vi "Fractional-octave Analysis with IC (peak mode).vi"(0 "scaled signal [EU]":dbl[](array[numeric]) format="%.2f", 1 "peak detection mode":T1(ring), 2 "filter bank parameters":T2 {"standard filter bandwidth" format="%.2f"; "special filter bandwidth" format="%.2f"; "lowpass filter coefficients"."Forward Coefficients" format="%.2f"; "lowpass filter coefficients"."Reverse Coefficients" format="%.2f"; "standard filter coefficients"."Forward Coefficients" format="%.2f"; "standard filter coefficients"."Reverse Coefficients" format="%.2f"; "special filter coefficients"."Forward Coefficients" format="%.2f"; "special filter coefficients"."Reverse Coefficients" format="%.2f"}, 3 "internal filter state IN":T3 {"linear averaging"."size" format="%.2f"; "linear averaging"."squared sum" format="%.2f"; "exponential averaging"."peak detector" format="%.2f"; "exponential averaging"."exponential averaging" format="%.2f"; "result" format="%.2f"; "lowpass filter" format="%.2f"; "octave filter"."Octave filter" format="%.2f"}, 4 "reset peak detection (F)":bool, 5 "filter init/cont (init:F)":bool) -> (6 "peak band power [EU^2 rms]":dbl[](array[numeric]) format="%.2f", 7 "settled?":bool, 8 "internal filter state OUT":T3 {"linear averaging"."size" format="%.2f"; "linear averaging"."squared sum" format="%.2f"; "exponential averaging"."peak detector" format="%.2f"; "exponential averaging"."exponential averaging" format="%.2f"; "result" format="%.2f"; "lowpass filter" format="%.2f"; "octave filter"."Octave filter" format="%.2f"})   [LabVIEW 2017]
doc: "Performs a peak fractional-octave analysis on the input signal. This VI requires the filter bank parameters and initialize filter state information the Design Octave Filter Set VI generates.\nThis VI returns the peak power in each fractional-octave band.\nThe internal filter state IN and internal filter state OUT keep track of the internal state of the filter to ensure continuous operation of the filter. To achieve this continuous operation, you must call this VI the first time with filter init/cont set to FALSE. Call it all subsequent times with filter init/cont set to TRUE. Wire the internal filter state OUT of this call to the internal filter state IN for the next call to this VI."
uses:
  <vilib>/addons/Sound and Vibration/svt_Octave/SoundVib_Octave.lvlib
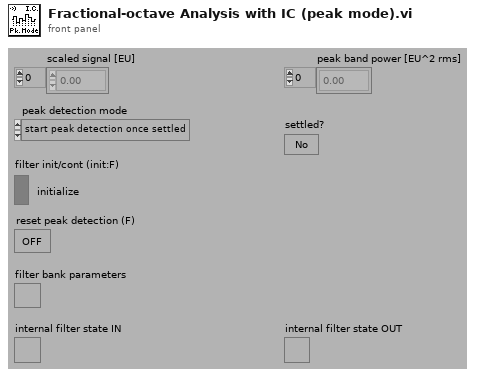
[diagram p1: front panel]
types:
  T1 = enum16{"start peak detection once settled", "continuous peak detection", "single peak detection"}
  T2 = cluster{"# special filters":i32, "special filter coefficients":cluster{"filter structure":enum32{"IIR 2nd Order", "IIR 4th Order"}, "Reverse Coefficients":dbl[], "Forward Coefficients":dbl[]}[], "# filters per octave":cluster{"# filters":i32, "starting at":i32}[], "standard filter coefficients":cluster{"filter structure":enum32{"IIR 2nd Order", "IIR 4th Order"}, "Reverse Coefficients":dbl[], "Forward Coefficients":dbl[]}[], "# decimation steps":i32, "lowpass filter coefficients":cluster{"filter structure":enum32{"IIR 2nd Order", "IIR 4th Order"}, "Reverse Coefficients":dbl[], "Forward Coefficients":dbl[]}, "# samples to settle":i32, "special filter bandwidth":dbl[], "standard filter bandwidth":dbl[]}
  T3 = cluster{"octave filter":cluster{"Octave filter":dbl[]}[], "decimation":i32[], "lowpass filter":dbl[][], "exponential averaging":cluster{"exponential averaging":dbl, "peak detector":dbl}[], "linear averaging":cluster{"squared sum":dbl, "size":dbl}[], "result":dbl[], "# samples since init":i32}
  T4 = cluster{"octave filter":cluster{"Octave filter":dbl[]}[], "decimation":i32[], "lowpass filter":dbl[][], "exponential averaging":cluster{"exponential averaging":dbl, "peak detector":dbl}[], "linear averaging":cluster{"squared sum":dbl, "size":dbl}[], "result":dbl[], "# samples since init":u64}
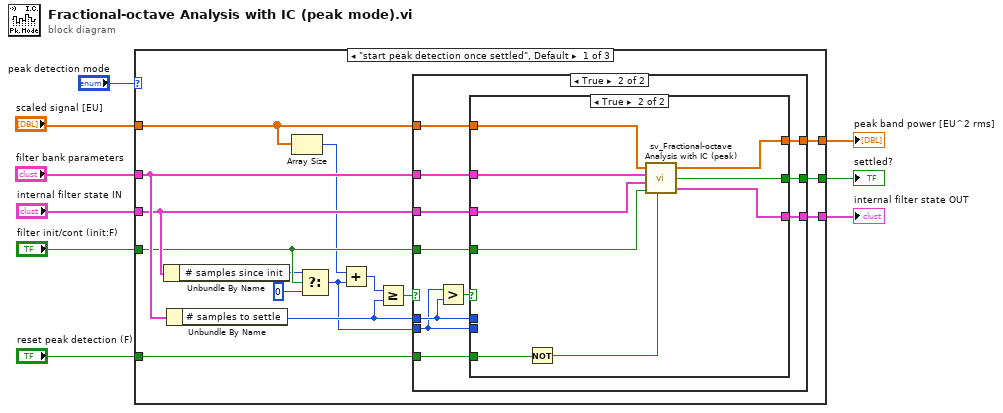
[diagram p0: block diagram]
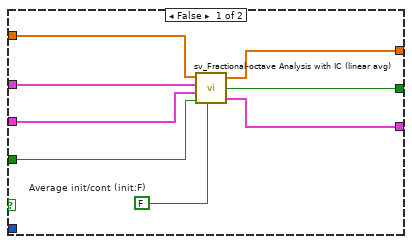
[diagram p2: hidden frame]
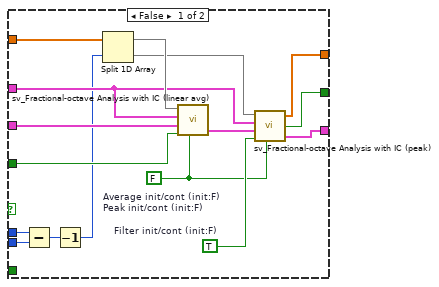
[diagram p3: hidden frame]
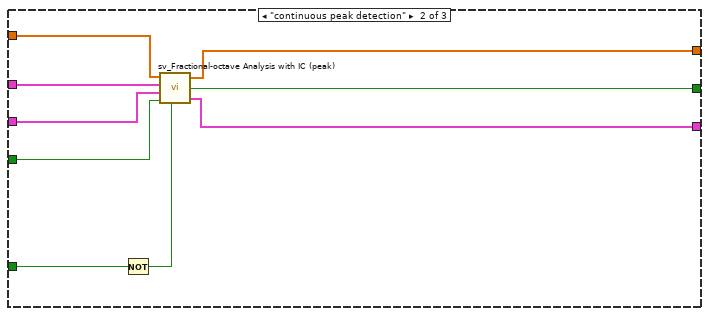
[diagram p4: hidden frame]
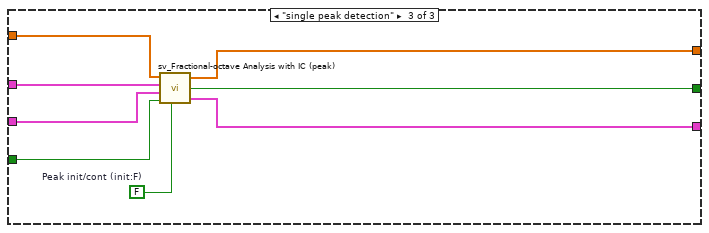
[diagram p5: hidden frame]
diagram:
  n1 = case shown="\"start peak detection once settled\", Default" "peak detection mode" {
    tunnel: "scaled signal [EU]" -> [w18 w77 w85]
    tunnel: "filter bank parameters" -> [w24 w76 w84]
    tunnel: "internal filter state IN" -> [w23 w75 w83]
    tunnel: "filter init/cont (init:F)" -> [w20 w74 w82]
    tunnel: [w13 w73 w80] -> w4
    tunnel: [w12 w72 w79] -> w3
    tunnel: [w11 w71 w78] -> w2
    tunnel: "reset peak detection (F)" -> [w10 w70 _]
    frame "start peak detection once settled", Default {
      n2 = Unbundle By Name(w23) -> ("# samples since init"=w19:i32)
      n3 = Unbundle By Name(w24) -> ("# samples to settle"=w22:i32)
      n4 = Array Size(array=w18) -> (size(s)=w16:i32)
      n5 = Select(t=w19, s=w20, f=0) -> (s? t:f=w14:i32)
      n6 = Add(x=w16, y=w14) -> (x+y=w15:i32)
      n7 = Greater Or Equal?(x=w15, y=w22) -> (x >= y?=w21:bool)
      n8 = case shown="True" w21 {
        tunnel: w24 -> [w32 w43]
        tunnel: w18 -> [w31 w40]
        tunnel: w23 -> [w29 w42]
        tunnel: w20 -> [w28 w41]
        tunnel: w22 -> [_ w38]
        tunnel: w14 -> [_ w37]
        tunnel: [w27 w36] -> w13
        tunnel: [w26 w35] -> w12
        tunnel: [w25 w34] -> w11
        tunnel: w10 -> [_ w33]
        frame False {
          w30 = FALSE  # Average init/cont (init:F)
          n9 = call <vilib>:"sv_Fractional-octave Analysis with IC (linear avg).vi"("scaled signal [EU]"=w31, "filter bank parameters"=w32, "internal filter state IN"=w29, "average init/cont (cont:T)"=w30, "filter init/cont (init:F)"=w28) -> ("linear avg band power [EU^2 rms]"=w27:dbl[], "settled?"=w26:bool, "internal filter state OUT"=w25:T4)  [unwired: 1 in]
        }
        frame True {
          n10 = Greater?(x=w37, y=w38) -> (0:w39:bool)
          n11 = case shown="True" w39 {
            tunnel: w43 -> [w49 w68]
            tunnel: w42 -> [w54 w67]
            tunnel: w41 -> [w53 w66]
            tunnel: w40 -> [w59 w65]
            tunnel: w38 -> [w58 _]
            tunnel: w37 -> [w57 _]
            tunnel: [w47 w64] -> w36
            tunnel: [w46 w63] -> w35
            tunnel: [w45 w62] -> w34
            tunnel: w33 -> [_ w61]
            frame False {
              w52 = TRUE  # Filter init/cont (init:F)
              w48 = FALSE  # Average init/cont (init:F) Peak init/cont (init:F)
              n12 = Subtract(x=w58, y=w57) -> (x-y=w56:i32)
              n13 = Decrement(x=w56) -> (x-1=w44:i32)
              n14 = Split 1D Array(array=w59, index=w44) -> (first subarray=w55:dbl[], second subarray=w51:dbl[])
              n15 = call <vilib>:"sv_Fractional-octave Analysis with IC (linear avg).vi"("scaled signal [EU]"=w55, "filter bank parameters"=w49, "internal filter state IN"=w54, "average init/cont (cont:T)"=w48, "filter init/cont (init:F)"=w53) -> ("internal filter state OUT"=w50:T4)  [unwired: 1 in, 2 out]
              n16 = call <vilib>:"sv_Fractional-octave Analysis with IC (peak).vi"("scaled signal [EU]"=w51, "filter bank parameters"=w49, "internal filter state IN"=w50, "peak init/cont (init:F)"=w48, "filter init/cont (init:F)"=w52) -> ("peak band power [EU^2 rms]"=w47:dbl[], "settled?"=w46:bool, "internal filter state OUT"=w45:T4)  [unwired: 1 in]
            }
            frame True {
              n17 = Not(x=w61) -> (.not. x?=w60:bool)
              n18 = call <vilib>:"sv_Fractional-octave Analysis with IC (peak).vi"("scaled signal [EU]"=w65, "filter bank parameters"=w68, "internal filter state IN"=w67, "peak init/cont (init:F)"=w60, "filter init/cont (init:F)"=w66) -> ("peak band power [EU^2 rms]"=w64:dbl[], "settled?"=w63:bool, "internal filter state OUT"=w62:T4)  [unwired: 1 in]
            }
          }
        }
      }
    }
    frame "continuous peak detection" {
      n19 = Not(x=w70) -> (.not. x?=w69:bool)
      n20 = call <vilib>:"sv_Fractional-octave Analysis with IC (peak).vi"("scaled signal [EU]"=w77, "filter bank parameters"=w76, "internal filter state IN"=w75, "peak init/cont (init:F)"=w69, "filter init/cont (init:F)"=w74) -> ("peak band power [EU^2 rms]"=w73:dbl[], "settled?"=w72:bool, "internal filter state OUT"=w71:T4)  [unwired: 1 in]
    }
    frame "single peak detection" {
      w81 = FALSE  # Peak init/cont (init:F)
      n21 = call <vilib>:"sv_Fractional-octave Analysis with IC (peak).vi"("scaled signal [EU]"=w85, "filter bank parameters"=w84, "internal filter state IN"=w83, "peak init/cont (init:F)"=w81, "filter init/cont (init:F)"=w82) -> ("peak band power [EU^2 rms]"=w80:dbl[], "settled?"=w79:bool, "internal filter state OUT"=w78:T4)  [unwired: 1 in]
    }
  }
  "peak band power [EU^2 rms]" <- w4
  "internal filter state OUT" <- w2
  "settled?" <- w3
